vi "Untitled 1 (SubVI).vi"(9 "upper limit 2":dbl, 10 "upper limit":dbl, 11 "Throttle":dbl) -> (2 "Numeric 2":dbl, 3 "Numeric":dbl)   [LabVIEW 2015]
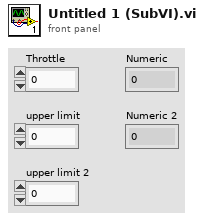
[diagram p1: front panel]
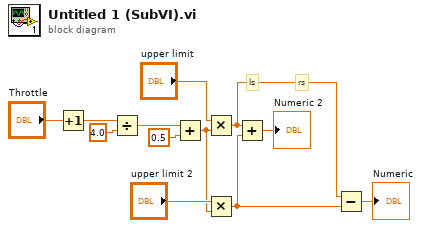
[diagram p0: block diagram]
diagram:
  # "rs"
  # "ls"
  n1 = Increment(x="Throttle") -> (x+1=w7:dbl)
  n2 = Divide(x=w7, y=4.0) -> (x/y=w5:dbl)
  n3 = Add(x=w5, y=0.5) -> (x+y=w8:dbl)
  n4 = Multiply(x="upper limit", y=w8) -> (x*y=w12:dbl)
  n5 = Multiply(x="upper limit 2", y=w8) -> (x*y=w10:dbl)
  n6 = Add(x=w12, y=w10) -> (x+y=→"Numeric 2":dbl)
  n7 = Subtract(x=w12, y=w10) -> (x-y=→"Numeric":dbl)
